vi "set Voxel Dimensions In Real Units.vi"(7 "pVoxelDepthInRealUnits":dbl, 9 "pVoxelHeightInRealUnits":dbl, 10 "pVoxelWidthInRealUnits":dbl, 11 "pSinkId":i32) -> (3 "function return":i32)   [LabVIEW 2012, in "cvlib.lvlib"]
doc: "extern \"C\"__declspec(dllexport) long __cdecl setVoxelDimensionsInRealUnits( long pSinkId,\n double pVoxelWidthInRealUnits,\n double pVoxelHeightInRealUnits,\n double pVoxelDepthInRealUnits);"
uses:
  cvlib.lvlib
  cvlib.dll
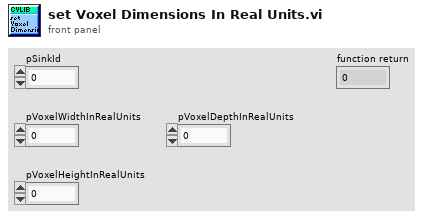
[diagram p1: front panel]
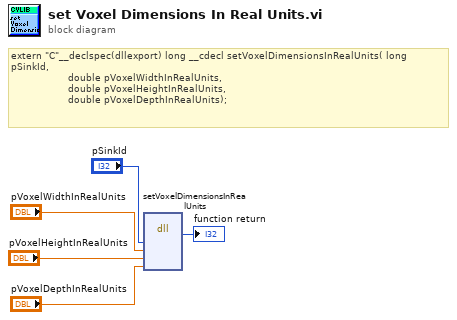
[diagram p0: block diagram]
diagram:
  # "extern \"C\"__declspec(dllexport) long __cdecl setVoxelDimensionsInRealUnits( long pSinkId,\n\t\t\t\t\t\t\t\t\t\t\t\t\t\t\t\t\t\t\tdouble pVoxelWidthInRealUnits,\n\t\t\t\t\t\t\t\t\t\t\t\t\t\t\t\t\t\t\tdouble pVoxelHeightInRealUnits,\n\t\t\t\t\t\t\t\t\t\t\t\t\t\t\t\t\t\t\tdouble pVoxelDepthInRealUnits);"
  n1 = dll-call lib="C:/Users/myerslab/workspace2/Libraries/ClearVolume/cpp/labview/lvcvlib/cvlib.*" fn="setVoxelDimensionsInRealUnits"("pSinkId"="pSinkId", "pVoxelWidthInRealUnits"="pVoxelWidthInRealUnits", "pVoxelHeightInRealUnits"="pVoxelHeightInRealUnits", "pVoxelDepthInRealUnits"="pVoxelDepthInRealUnits") -> (→"function return":i32)  [unwired: 7 in, 2 out]
